vi "PI_Start_Wave_Gen.vi"(0 "System no.":i32, 11 "error in":errorcluster, 12 "Axis":i32, 13 "Line Scan":bool) -> (4 "System no. (dup)":i32, 15 "error out":errorcluster)   [LabVIEW 2011]
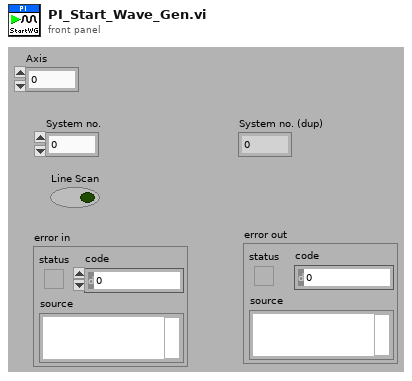
[diagram p1: front panel]
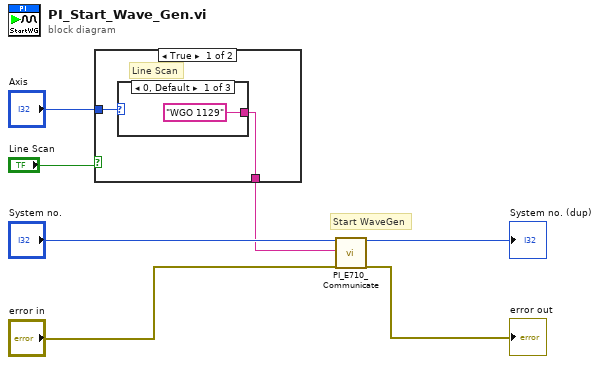
[diagram p0: block diagram]
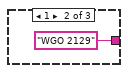
[diagram p2: hidden frame]
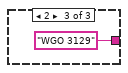
[diagram p3: hidden frame]
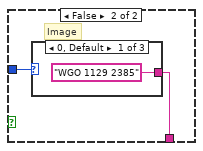
[diagram p4: hidden frame]
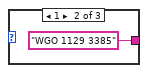
[diagram p5: hidden frame]
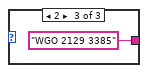
[diagram p6: hidden frame]
diagram:
  # "Start WaveGen"
  n1 = case shown="True" "Line Scan" {
    tunnel: "Axis" -> [w9 w14]
    tunnel: [w8 w13] -> w3
    frame True {
      # "Line Scan"
      n2 = case shown="0, Default" w9 {
        tunnel: ["WGO 1129" ("String to send") "WGO 2129" ("String to send") "WGO 3129" ("String to send")] -> w8
        frame 0, Default {
        }
        frame 1 {
        }
        frame 2 {
        }
      }
    }
    frame False {
      # "Image"
      n3 = case shown="0, Default" w14 {
        tunnel: ["WGO 1129 2385" ("String to send") "WGO 1129 3385" ("String to send") "WGO 2129 3385" ("String to send")] -> w13
        frame 0, Default {
        }
        frame 1 {
        }
        frame 2 {
        }
      }
    }
  }
  n4 = call "PI_E710_Communicate.vi"("System no."="System no.", "String to send"=w3, "error in"="error in") -> ("System no. (dup)"=→"System no. (dup)":i32, "error out"=→"error out":errorcluster)  [unwired: 14 in, 1 out]
